vi "niRFUtil RFHS Channelizer ClearFineTuneResampler CSG.vi"(0 "Resampler Ref":refnum<data-value>, 11 "error in (no error)":errorcluster) -> (6 "Data Left":csg[](array[numeric]), 15 "error out":errorcluster)   [LabVIEW 2015, in "niRFUtil.lvlib"]
uses:
  niRFUtil.lvlib
  Includes/niRFUtil RFHS Channelizer ResamplerInfo CSG.ctl
  Includes/niRFUtil RFHS Channelizer FilterRef.ctl
  Includes/niRFUtil RFHS Channelizer ChannelizerBufferingMode.ctl
  Utilities/Data FIFO/niRFUtil RFHS FIFO Reference.ctl
  Utilities/Data FIFO/niRFUtil RFHS FIFO.ctl
  Includes/niRFUtil RFHS Channelizer ChannelizerFlags.ctl
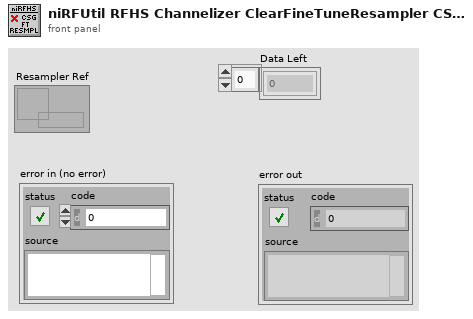
[diagram p1: front panel]
types:
  T1 = typedef "niRFUtil.lvlib/niRFUtil RFHS Channelizer ResamplerInfo CSG.ctl" = cluster{"Filter LVRef":T2, "Mode":T3, "History":csg[], "Buffer":csg[], "FIFO":T4, "BufferW":u32, "BufferR":u32, "Phase":dbl, "Flags":T6, "Reset Cnt":i64}
  T2 = typedef "niRFUtil.lvlib/niRFUtil RFHS Channelizer FilterRef.ctl" = cluster{"Ref":u64, "GUID":u64, "Upsample":i32, "Downsample":i32, "Size":i32, "Num Taps":i32}
  T3 = typedef "niRFUtil.lvlib/niRFUtil RFHS Channelizer ChannelizerBufferingMode.ctl" = enum32{"Unbuffered", "Finite", "Continuous"}
  T4 = typedef "niRFUtil.lvlib/niRFUtil RFHS FIFO Reference.ctl" = cluster{"Read Lock":refnum<data-value>, "Info":T5, "Write Lock":refnum<data-value>}
  T5 = typedef "niRFUtil.lvlib/niRFUtil RFHS FIFO.ctl" = cluster{"ID":u64, "Length":u32}
  T6 = typedef "niRFUtil.lvlib/niRFUtil RFHS Channelizer ChannelizerFlags.ctl" = u32
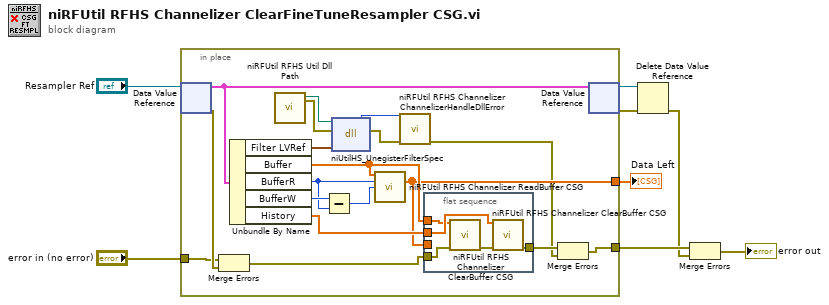
[diagram p0: block diagram]
diagram:
  n1 = in-place {
    in-place-border: [w18] -> w7
    in-place-border: "error in (no error)" -> [w16]
    in-place-border: [w11] -> w4
    n2 = in-place-dvr #1("Resampler Ref") -> (w24:T1, w17:errorcluster)
    n3 = Merge Errors(w16, w17) -> (w15:errorcluster)
    n4 = Unbundle By Name(w24) -> ("Filter LVRef"=w25:T2, "Buffer"=w19:csg[], "BufferR"=w22:u32, "BufferW"=w23:u32, "History"=w20:csg[])
    n5 = call "niRFUtil RFHS Util Dll Path.vi"() -> ("error out"=w9:errorcluster, "Path"=w26:path)  [unwired: 7 in, 3 out]
    n6 = Subtract(x=w23, y=w22) -> (x-y=w21:u32)
    n7 = dll-call lib="?" fn="niUtilHS_UnegisterFilterSpec"(path in=w26, error in=w9, "lvRef"=w25) -> (error out=w14:errorcluster, "return type"=w13:i32)  [unwired: 2 in, 1 out]
    n8 = call "niRFUtil RFHS Channelizer ReadBuffer CSG.vi"("Buffer"=w19, "Index"=w22, "Length"=w21) -> ("Data"=w18:csg[])  [unwired: 12 in]
    n9 = call "niRFUtil RFHS Channelizer ChannelizerHandleDllError.vi"("Error"=w13, "error in (no error)"=w14) -> ("error out"=w10:errorcluster)  [unwired: 13 in]
    n10 = flat-sequence {
      tunnel: w20 -> [w30]
      tunnel: w19 -> [w29]
      tunnel: w18 -> [_]
      tunnel: w15 -> [w28]
      tunnel: [w27] -> w12
      frame #0 {
        n11 = call "niRFUtil RFHS Channelizer ClearBuffer CSG.vi"("Buffer"=w29, "error in (no error)"=w28) -> ("error out"=w31:errorcluster)  [unwired: 13 in]
        n12 = call "niRFUtil RFHS Channelizer ClearBuffer CSG.vi"("Buffer"=w30, "error in (no error)"=w31) -> ("error out"=w27:errorcluster)  [unwired: 13 in]
      }
    }
    n13 = Merge Errors(w12, w10) -> (w11:errorcluster)
    n14 = in-place-dvr #1(w24) -> (w8:refnum<data-value>, w3:errorcluster)
  }
  "Data Left" <- w7
  n15 = Delete Data Value Reference(data value reference=w8, error in=w3) -> (error out=w2:errorcluster)  [unwired: 1 out]
  n16 = Merge Errors(w4, w2) -> (→"error out":errorcluster)
